vi "DCIR_Create.vi"(0 "reference in":refnum<class "DCIR.lvclass">, 5 "DCIR Parameters":T1={"Pulse Mode"=2, "Initial SoC (%)"=650.0, "Pulse Current (A)"=1000.0, "Pulse Duration (S)"=500.0} {"Pulse Mode" items=["Discharge"=1, "Charge"=2]; "Initial SoC (%)" min=0.0 max=100.0}, 7 "Logger":refnum<class "Logger.lvclass">, 9 "HPS17K Refs":refnum<class "HPS-17000.lvclass">[](array[class]), 11 "Error In":errorcluster) -> (4 "reference out":refnum<class "DCIR.lvclass">, 6 "ProcessViRef":refnum<vi>, 15 "Error Out":errorcluster)   [LabVIEW 2023, in "DCIR.lvclass"]
uses:
  DCIR.lvclass
  DCIR.lvclass/DCIR.ctl
  Logger_class/Logger.lvclass
  <instrlib>/HPS-17000/HPS-17000.lvclass
  Types/DCIR Mode.ctl
  Types/DCIR Parameters.ctl
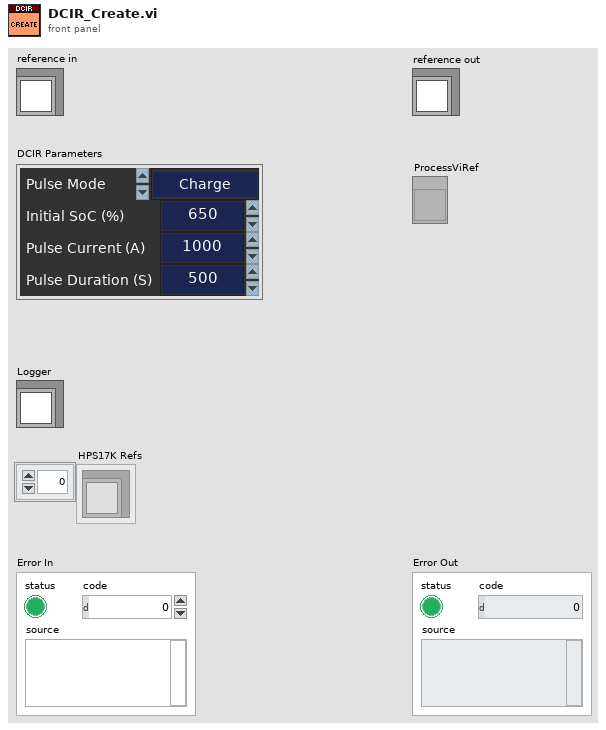
[diagram p1: front panel]
types:
  T1 = typedef "DCIR Parameters.ctl" = cluster{"Pulse Mode":T2, "Initial SoC (%)":dbl, "Pulse Current (A)":dbl, "Pulse Duration (S)":dbl}
  T2 = typedef "DCIR Mode.ctl" = u16
  T3 = typedef "DCIR.lvclass/ObjectAttributes.ctl" = cluster{"DCIR Parameters":T1, "Logger":refnum<class "Logger.lvclass">, "HPS17K Refs":refnum<class "HPS-17000.lvclass">[]}
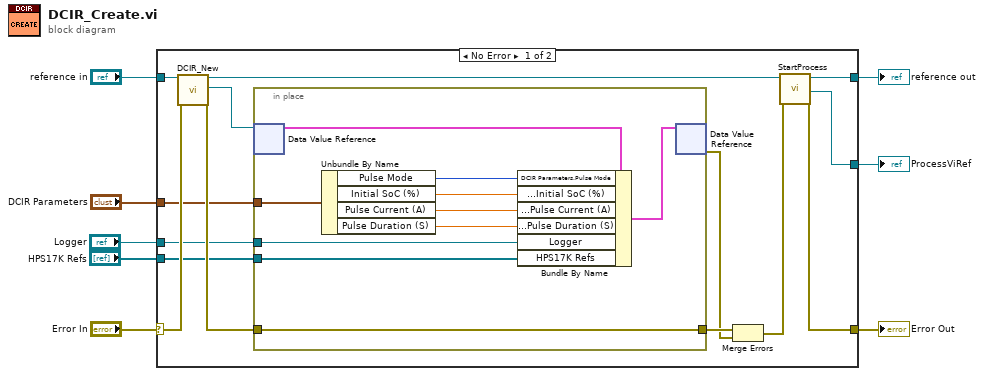
[diagram p0: block diagram]
diagram:
  n1 = case shown="No Error" "Error In" {
    selector: "Error In" -> [w21 w34]
    tunnel: [w15 w34] -> w7
    tunnel: "reference in" -> [w22 w33]
    tunnel: [w17 w33] -> w5
    tunnel: [w14 _] -> w4
    tunnel: "DCIR Parameters" -> [w13 _]
    tunnel: "Logger" -> [w10 _]
    tunnel: "HPS17K Refs" -> [w9 _]
    frame No Error {
      n2 = call "DCIR_New.vi"("reference in"=w22, "Error In"=w21) -> ("reference out"=w18:refnum<class "DCIR.lvclass">, "DVRRefOut"=w12:refnum<data-value>, "Error Out"=w20:errorcluster)  [unwired: 14 in, 1 out]
      n3 = in-place {
        in-place-border: w20 -> [w32]
        in-place-border: [w32] -> w19
        in-place-border: w13 -> [w29]
        in-place-border: w10 -> [w28]
        in-place-border: w9 -> [w27]
        n4 = in-place-dvr #1(w12) -> (w31:T3)  [unwired: 1 out]
        n5 = Unbundle By Name(w29) -> ("Pulse Mode"=w26:T2, "Initial SoC (%)"=w25:dbl, "Pulse Current (A)"=w24:dbl, "Pulse Duration (S)"=w23:dbl)
        n6 = Bundle By Name(cluster=w31, "DCIR Parameters.Pulse Mode"=w26, "DCIR Parameters.Initial SoC (%)"=w25, "DCIR Parameters.Pulse Current (A)"=w24, "DCIR Parameters.Pulse Duration (S)"=w23, "Logger"=w28, "HPS17K Refs"=w27) -> (w30:T3)
        n7 = in-place-dvr #1(w30) -> (w11:errorcluster)  [unwired: 1 out]
      }
      n8 = Merge Errors(w19, w11) -> (w16:errorcluster)
      n9 = call "StartProcess.vi"("reference in"=w18, "Error In"=w16) -> ("reference out"=w17:refnum<class "DCIR.lvclass">, "ProcessViRef"=w14:refnum<vi>, "Error Out"=w15:errorcluster)  [unwired: 13 in, 2 out]
    }
    frame Error {
      # "VI-TechBaseTemplate_Simple_6x8x6"
    }
  }
  "Error Out" <- w7
  "reference out" <- w5
  "ProcessViRef" <- w4
